vi "DVR Flatten.vi"(7 "payload in":u8[](array[numeric]), 8 "error in (no error)":errorcluster, 9 "FIFO Timestamps":T1, 10 "Data In":refnum<data-value>[](array[refnum]), 11 "CIFChannels in":refnum<class "CIFChannels.lvclass">) -> (0 "error out":errorcluster, 1 "Total Length":i32, 2 "Data Out":refnum<data-value>[](array[refnum]), 3 "CIFChannels out":refnum<class "CIFChannels.lvclass">, 5 "payload out":u8[](array[numeric]))   [LabVIEW 2021, in "CIF_NIChn_FIFO_DAQ_DVR.lvclass"]
uses:
  CIF_NIChn_FIFO_DAQ_DVR.lvclass
  ChannelCommon/typedef/Datatype Waveform.ctl
  ChannelCommon/typedef/TimeStamps.ctl
  CIFChannels/CIFChannels.lvclass
  CIFChannels/CIFChannels.lvclass/CIFChannels.ctl
  <vilib>/CIF Foundation/CIF Utilities/DataTypes/Endian.ctl
  ChannelCommon/Utilities/Flatten Header.vi
  CIFChannels/Utilities/Update FIFO Header.vi
  <vilib>/CIF Foundation/CIF Utilities/DataTypes/Flatten I64.vi
  <vilib>/CIF Foundation/CIF Utilities/Time/System Time/Get System Time.vi
  <vilib>/CIF Foundation/CIF Utilities/Time/System Time/LabVIEW Time to TAI Time.vi
  CIF_NIChn_FIFO_DAQ_DVR.lvclass/CIF_NIChn_FIFO_DAQ_DVR.ctl
  <vilib>/CIF Foundation/CIF Utilities/DataTypes/DataTypes_CIF_U.lvlib
  ChannelCommon/ChannelCommon.lvlib
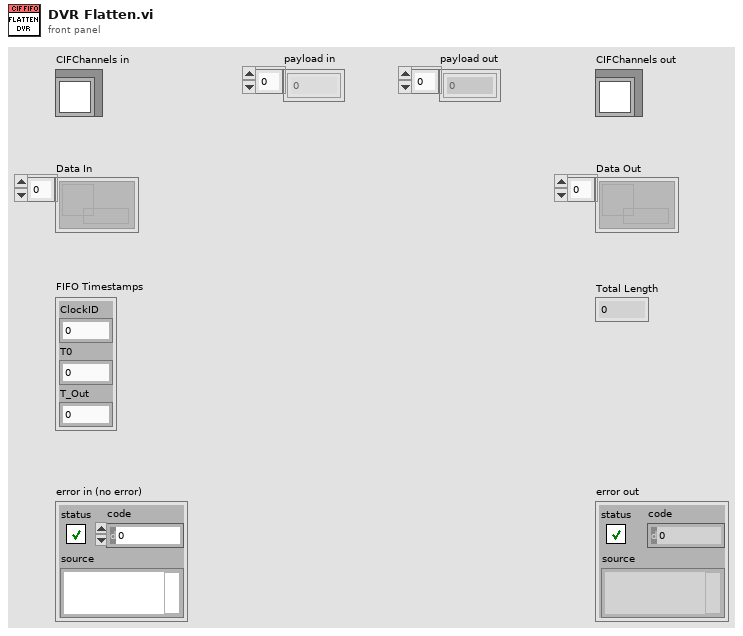
[diagram p1: front panel]
types:
  T1 = typedef "ChannelCommon.lvlib/TimeStamps.ctl" = cluster{"ClockID":u8, "T0":i64, "T_Out":i64}
  T2 = typedef "DataTypes_CIF_U.lvlib/Endian.ctl" = enum16{"Little Endian", "Big Endian"}
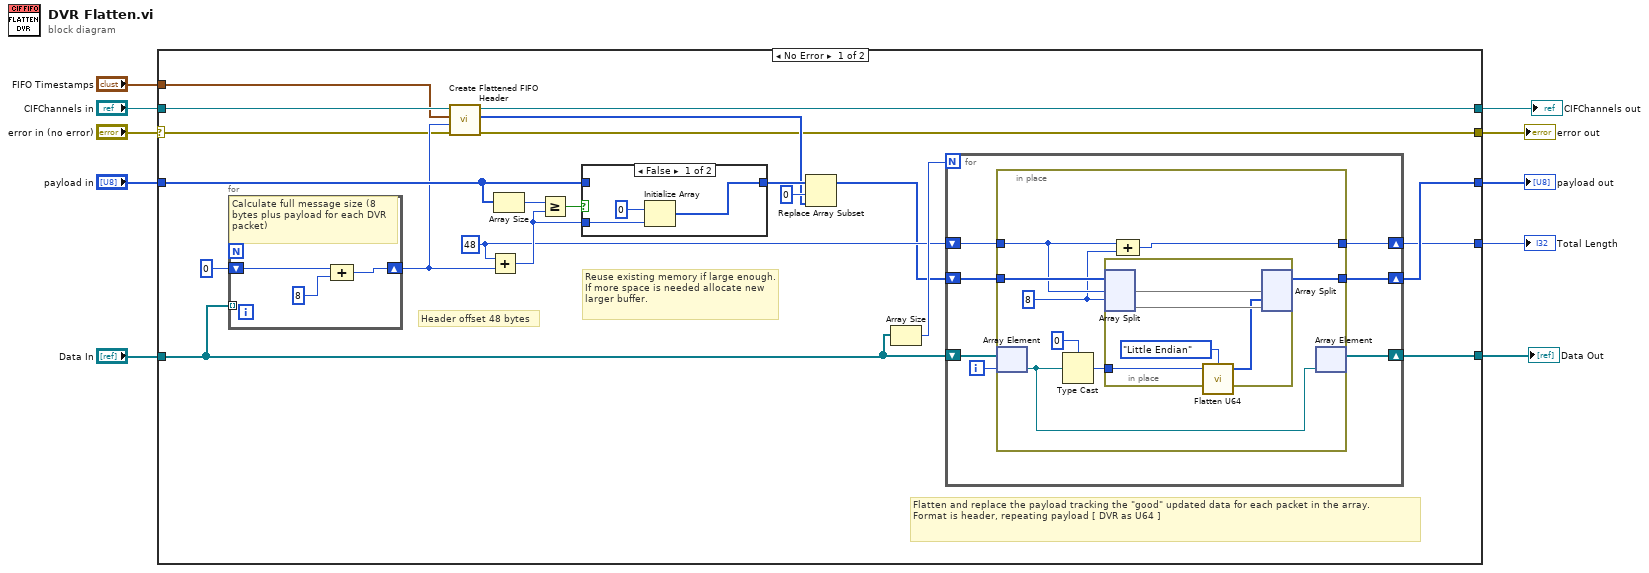
[diagram p0: block diagram]
diagram:
  n1 = case shown="No Error" "error in (no error)" {
    selector: "error in (no error)" -> [w12 w62]
    tunnel: [w11 w62] -> w9
    tunnel: "Data In" -> [w21 w59]
    tunnel: "CIFChannels in" -> [w18 w61]
    tunnel: [w15 w61] -> w1
    tunnel: [w26 w60] -> w8
    tunnel: "payload in" -> [w28 w60]
    tunnel: [w25 w59] -> w4
    tunnel: [w23 _] -> w6
    tunnel: "FIFO Timestamps" -> [w17 _]
    frame No Error {
      w24 = 48 ("y")
      # "Flatten and replace the payload tracking the \"good\" updated data for each packet in the array.\nFormat is header, repeating payload [ DVR as U64 ]"
      # "Header offset 48 bytes"
      # "Reuse existing memory if large enough.  If more space is needed allocate new larger buffer."
      n2 = for {
        tunnel: w21 -> [_] mode=indexing
        shift-right: [w34] -> w13
        shift-left: 0 -> [w33]
        # "Calculate full message size (8 bytes plus payload for each DVR packet)"
        n3 = Compound Arithmetic op=ADD(w33, 8 ("value")) -> (w34:i32)
      }
      n4 = call "Create Flattened FIFO Header.vi"("error in (no error)"=w12, "Data Length"=w13, "FIFO Timestamps"=w17, "CIFChannels in"=w18) -> ("error out"=w11:errorcluster, "Flattened FIFO Header"=w14:u8[], "CIFChannels out"=w15:refnum<class "CIFChannels.lvclass">)  [unwired: 5 in]
      n5 = Add(x=w24, y=w13) -> (x+y=w29:i32)
      n6 = Array Size(array=w28) -> (size(s)=w31:i32)
      n7 = Greater Or Equal?(x=w31, y=w29) -> (x >= y?=w30:bool)
      n8 = case shown="False" w30 {
        tunnel: w28 -> [_ w58]
        tunnel: [w55 w58] -> w16
        tunnel: w29 -> [w57 _]
        frame False {
          n9 = Initialize Array(u8 0, w57) -> (w55:u8[])
        }
        frame True {
        }
      }
      n10 = Replace Array Subset(array=w16, new element=w14, index=0) -> (w20:u8[])
      n11 = Array Size(array=w21) -> (size(s)=w27:i32)
      n12 = for {
        N: w27 -> [_]
        shift-right: [w40] -> w26
        shift-left: w20 -> [w41]
        shift-right: [w38] -> w23
        shift-left: w24 -> [w39]
        shift-right: [w35] -> w25
        shift-left: w21 -> [w37]
        i -> [w36]
        n13 = in-place {
          in-place-border: w41 -> [w49]
          in-place-border: [w48] -> w40
          in-place-border: w39 -> [w47]
          in-place-border: [w46] -> w38
          w45 = 8 ("value")
          n14 = in-place-array #1(w37, w36) -> (w42:refnum<data-value>)
          n15 = Type Cast(type=u64 0, x=w42) -> (*(type *) &x=w43:u64)
          n16 = in-place {
            in-place-border: w43 -> [w52]
            n17 = in-place-split #2(w49, w47, w45) -> (w54:u8[], w53:u8[])  [unwired: 1 out]
            n18 = call <vilib>:"Flatten U64.vi"("U64"=w52, "Endian"=Endian."Little Endian") -> ("Flat Data"=w51:u8[])  [unwired: 3 in]
            n19 = in-place-split #2(w54, w51, w53) -> (w48:u8[])  [unwired: 2 out]
          }
          n20 = Compound Arithmetic op=ADD(w47, w45) -> (w46:i32)
          n21 = in-place-array #1(w42) -> (w35:refnum<data-value>[])  [unwired: 1 out]
        }
      }
    }
    frame Error {
    }
  }
  "error out" <- w9
  "payload out" <- w8
  "Total Length" <- w6
  "Data Out" <- w4
  "CIFChannels out" <- w1
